vi "Renishaw-XL80_GetEC10Status.vi"(8 "error in (no error)":errorcluster, 11 "Renishaw-XL80_EMU in":refnum<class "Renishaw-XL80_EMU.lvclass">) -> (0 "error out":errorcluster, 2 "EC10Status":i32(ring) items=["EC10_CONNECTED"=0, "EC10_NOT_RESPONDING"=65536], 3 "Renishaw-XL80_EMU out":refnum<class "Renishaw-XL80_EMU.lvclass">)   [LabVIEW 2024, in "Renishaw-XL80_EMU.lvclass"]
doc: "This read only property returns the current status of the EC10. It indicates whether or not the EC10 is responding.\n\nDefinition\nHRESULT\nget_EC10Status(\n [out, retval] EC10_STATUS_CODES* pVal\n);\n\nParameters\npVal\nA variable that will be set one of the EC10_STATUS_CODES.\n\nComments\nThis property will return with an HRESULT of E_FAIL if the client has not previously connected to a DX10 by calling Connect.\n\nThe property will normally return an HRESULT of S_OK. However, it will return E_POINTER if the client supplies a null pointer for pVal.\n\nNote: if there is a XL laser connected to the DX10Adaptor COM interface this property returns the status of the associated XC device"
uses:
  Renishaw-XL80_EMU.lvclass
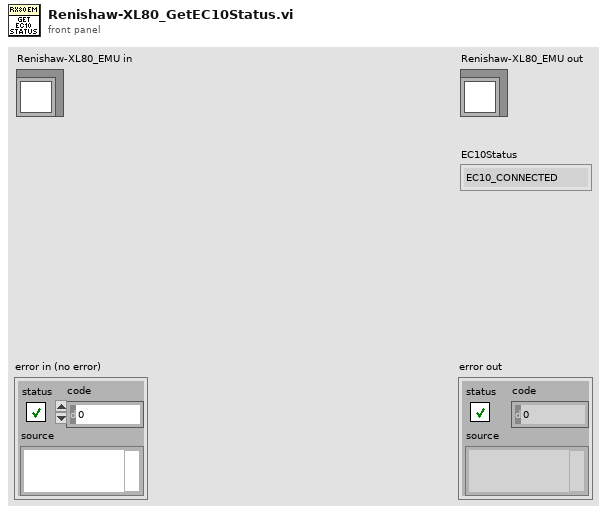
[diagram p1: front panel]
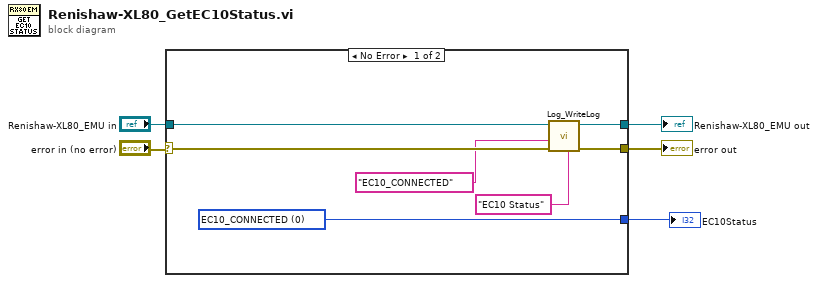
[diagram p0: block diagram]
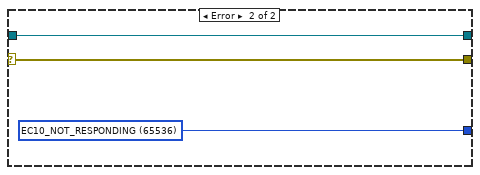
[diagram p2: hidden frame]
diagram:
  n1 = case shown="No Error" "error in (no error)" {
    selector: "error in (no error)" -> [w8 w14]
    tunnel: "Renishaw-XL80_EMU in" -> [w11 w15]
    tunnel: [w10 w15] -> w4
    tunnel: [w9 w14] -> w2
    tunnel: [w12 w13] -> w1
    frame No Error {
      w12 = 0 items=["EC10_CONNECTED"=0, "EC10_NOT_RESPONDING"=65536] ("EC10Status")
      n2 = call-dynamic "Log_WriteLog.vi"("Additional text"="EC10 Status", "error in (no error)"=w8, "Response"="EC10_CONNECTED", "Log in"=w11) -> ("error out"=w9:errorcluster, "Log out"=w10:refnum<class "Renishaw-XL80_EMU.lvclass">)  [unwired: 6 in]
    }
    frame Error {
      w13 = 65536 items=["EC10_CONNECTED"=0, "EC10_NOT_RESPONDING"=65536] ("EC10Status")
    }
  }
  "error out" <- w2
  "Renishaw-XL80_EMU out" <- w4
  "EC10Status" <- w1
